vi "Set-control-enable-single.vi"(8 "error in (no error)":errorcluster, 9 "Enable?":bool, 10 "Control name":T1, 11 "Panes in":T2) -> (0 "error out":errorcluster, 3 "Panes out":T2)   [LabVIEW 2013, in "MaterialCharacterization.lvlib" / "MC-UI.lvclass"]
uses:
  MC-UI.lvclass
  Panes-reference.ctl
  Control-names.ctl
  MC-UI.lvclass/MC-UI.ctl
  Read Controls lib.vi
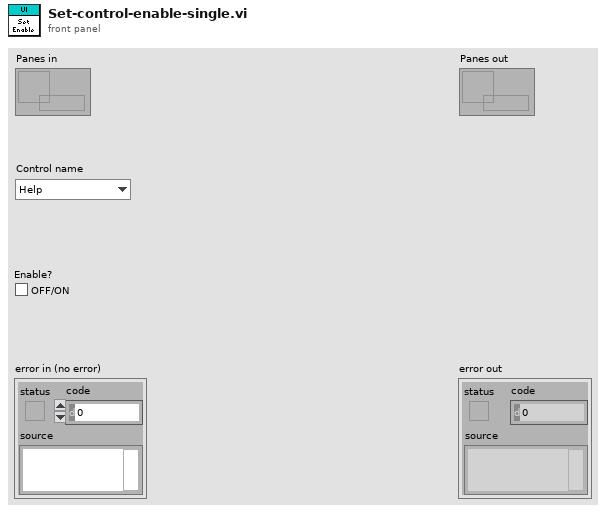
[diagram p1: front panel]
types:
  T1 = typedef "MaterialCharacterization.lvlib/MC-UI.lvclass/Control-names.ctl" = enum16{"Help", "Status", "Load configuration", "Save configuration", "Activate", "Start", "Stop", "Options"}
  T2 = typedef "MaterialCharacterization.lvlib/MC-UI.lvclass/Panes-reference.ctl" = refnum<data-value>
  T3 = enum8{"Enabled", "Disabled", "Disabled and Grayed Out"}
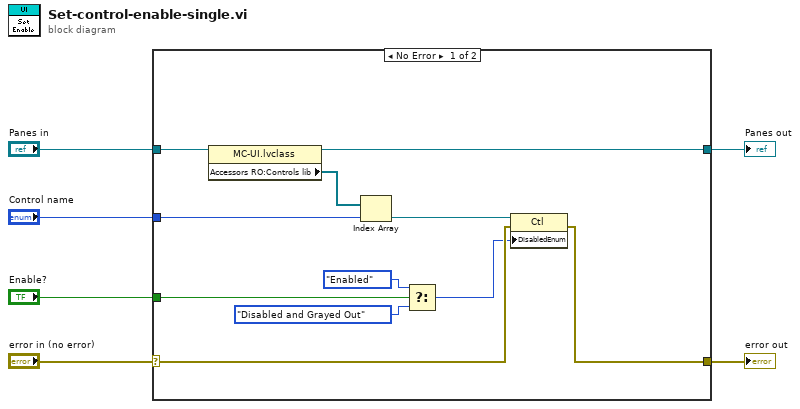
[diagram p0: block diagram]
diagram:
  n1 = case shown="No Error" "error in (no error)" {
    selector: "error in (no error)" -> [w11 w18]
    tunnel: [w14 w18] -> w5
    tunnel: [w13 w19] -> w3
    tunnel: "Panes in" -> [w17 w19]
    tunnel: "Control name" -> [w15 _]
    tunnel: "Enable?" -> [w10 _]
    frame No Error {
      n2 = property class="MC-UI.lvclass"(reference=w17) -> (reference out=w13:T2, "Accessors RO:Controls lib"=w16:refnum<vi>[])  [unwired: 1 in, 1 out]
      n3 = Index Array(array=w16, index=w15) -> (element=w12:refnum<vi>)
      n4 = Select(t=T3."Enabled" ("Disabled"), s=w10, f=T3."Disabled and Grayed Out" ("Disabled")) -> (s? t:f=w9:T3)
      n5 = property class="Ctl"(reference=w12, error in=w11, "DisabledEnum"=w9) -> (error out=w14:errorcluster)  [unwired: 1 out]
    }
    frame Error {
    }
  }
  "error out" <- w5
  "Panes out" <- w3
